vi "supergui create stop queue.vi"() -> (3 "STOP Queue out":refnum<queue>)   [LabVIEW 2013]
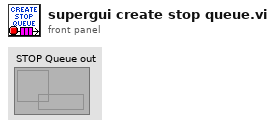
[diagram p1: front panel]
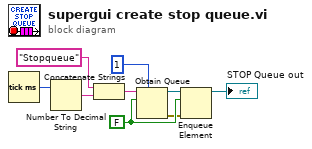
[diagram p0: block diagram]
diagram:
  w2 = FALSE
  n1 = Tick Count (ms)() -> (millisecond timer value=w5:u32)
  n2 = Number To Decimal String(number=w5) -> (decimal integer string=w6:string)  [unwired: 1 in]
  n3 = Concatenate Strings("Stopqueue" ("name (unnamed)"), w6) -> (w7:string)
  n4 = Obtain Queue(max queue size (-1, unlimited)=1, name (unnamed)=w7, element data type=w2) -> (queue out=w8:refnum<queue>, error out=w1:errorcluster)  [unwired: 2 in, 1 out]
  n5 = Enqueue Element(queue=w8, element=w2, error in (no error)=w1) -> (queue out=→"STOP Queue out":refnum<queue>)  [unwired: 1 in, 2 out]
